vi "USB2XXX_UART_WriteReadTest.vi"() -> ()   [LabVIEW 2010]
panel:
  in  "pConfig":T1={"BaudRate"=19200, "WordLength"=0, "StopBits"=0, "Parity"=0, "TEPolarity"=0}
  out "Readed Data Num":i32
  out "Read Data(Hex)":string
  in  "Write Data(Hex)":string="11 22 33 44 55 66 77 88"
  in  "Channel Index":u8(ring) items=["UART0", "UART1"]
  in  "Device Index":i32(ring) items=["0", "1", "2", "3", "4", "5"]
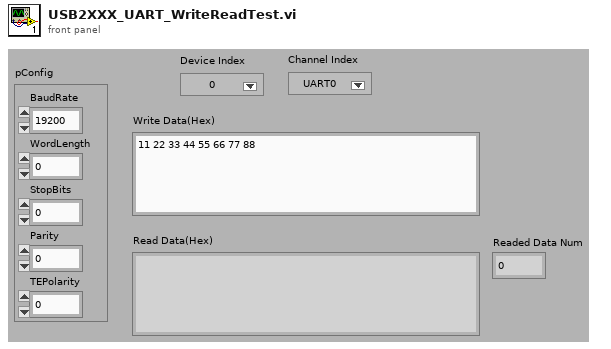
[diagram p1: front panel]
types:
  T1 = cluster{"BaudRate":u32, "WordLength":u8, "StopBits":u8, "Parity":u8, "TEPolarity":u8}
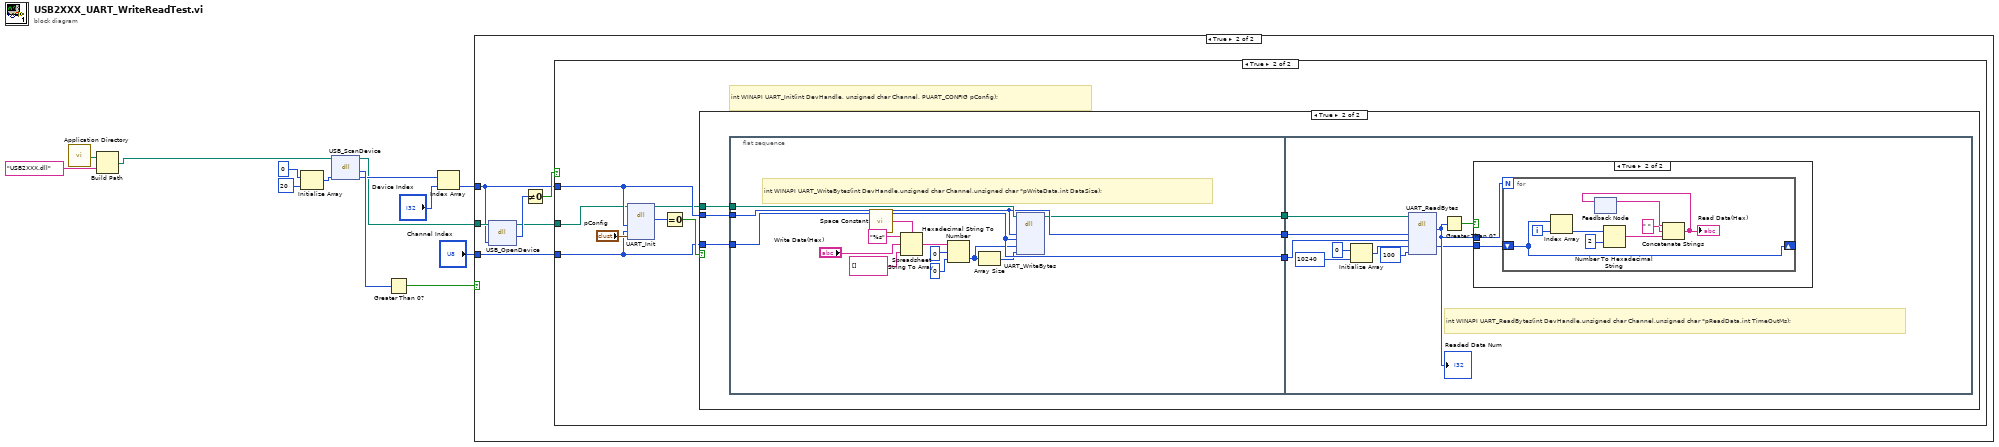
[diagram p0: block diagram]
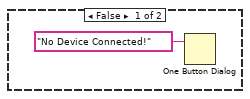
[diagram p2: hidden frame]
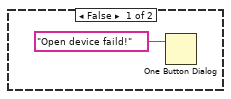
[diagram p3: hidden frame]
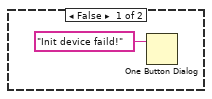
[diagram p4: hidden frame]
diagram:
  n1 = call <vilib>:"Application Directory.vi"() -> ("Application Directory"=w2:path)
  n2 = Build Path(base path=w2, name or relative path="USB2XXX.dll") -> (appended path=w1:path)
  n3 = Initialize Array(0, 20 ("dimension size")) -> (w11:i32[])
  n4 = dll-call lib="E:/OtherWork/STM32/USB2XXX_Example/examples/Labview/PublicFiles/USB2XXX.dll" fn="USB_ScanDevice"(path in=w1, "pDevNum"=w11) -> (path out=w6:path, "return type"=w10:i32, "pDevNum"=w9:i32[])  [unwired: 2 in, 1 out]
  n5 = Greater Than 0?(x=w10) -> (x > 0?=w7:bool)
  n6 = Index Array(array=w9, index="Device Index") -> (element=w5:i32)
  n7 = case shown="True" w7 {
    tunnel: w6 -> [_ w20]
    tunnel: w5 -> [_ w16]
    tunnel: "Channel Index" -> [_ w15]
    frame False {
      n8 = One Button Dialog(message="No Device Connected!") -> ()  [unwired: 1 in, 1 out]
    }
    frame True {
      n9 = dll-call lib="E:/OtherWork/STM32/USB2XXX_Example/examples/Labview/PublicFiles/USB2XXX.dll" fn="USB_OpenDevice"(path in=w20, "DevIndex"=w16) -> (path out=w17:path, "return type"=w19:u8)  [unwired: 3 in, 1 out]
      n10 = Not Equal To 0?(x=w19) -> (x != 0?=w18:bool)
      n11 = case shown="True" w18 {
        tunnel: w17 -> [_ w24]
        tunnel: w16 -> [_ w26]
        tunnel: w15 -> [_ w25]
        frame False {
          n12 = One Button Dialog(message="Open device faild!") -> ()  [unwired: 1 in, 1 out]
        }
        frame True {
          # "int WINAPI UART_Init(int DevHandle, unsigned char Channel, PUART_CONFIG pConfig);"
          n13 = dll-call lib="E:/OtherWork/STM32/USB2XXX_Example/sdk/api/Labview/USB2XXX.*" fn="UART_Init"(path in=w24, "DevHandle"=w26, "Channel"=w25, "pConfig"="pConfig") -> (path out=w23:path, "return type"=w22:i32)  [unwired: 5 in, 1 out]
          n14 = Equal To 0?(x=w22) -> (x = 0?=w28:bool)
          n15 = case shown="True" w28 {
            tunnel: w23 -> [_ w35]
            tunnel: w26 -> [_ w34]
            tunnel: w25 -> [_ w33]
            frame False {
              n16 = One Button Dialog(message="Init device faild!") -> ()  [unwired: 1 in, 1 out]
            }
            frame True {
              n17 = flat-sequence {
                tunnel: w35 -> [w41]
                tunnel: w34 -> [w40]
                tunnel: w33 -> [w39]
                tunnel: [w36] -> w32
                tunnel: [w40] -> w31
                tunnel: [w39] -> w30
                tunnel: w32 -> [w55]
                tunnel: w31 -> [w54]
                tunnel: w30 -> [w53]
                frame #0 {
                  # "int WINAPI UART_WriteBytes(int DevHandle,unsigned char Channel,unsigned char *pWriteData,int DataSize);"
                  n18 = call <vilib>:"Space Constant.vi"() -> ("String"=w44:string)
                  n19 = Spreadsheet String To Array(delimiter (Tab)=w44, format string="%s", spreadsheet string="Write Data(Hex)", array type (2D Dbl)=string[] []) -> (array=w47:string[])
                  n20 = Hexadecimal String To Number(string=w47, offset=0, default (0uL)=u8 0 ("default (0 U32)")) -> (number=w38:u8[])  [unwired: 1 out]
                  n21 = Array Size(array=w38) -> (size(s)=w37:i32)
                  n22 = dll-call lib="E:/OtherWork/STM32/USB2XXX_Example/sdk/api/Labview/USB2XXX.*" fn="UART_WriteBytes"(path in=w41, "DevHandle"=w40, "Channel"=w39, "pWriteData"=w38, "DataSize"=w37) -> (path out=w36:path)  [unwired: 7 in, 1 out]
                }
                frame #1 {
                  # "int WINAPI UART_ReadBytes(int DevHandle,unsigned char Channel,unsigned char *pReadData,int TimeOutMs);"
                  n23 = Initialize Array(u8 0 ("element"), 10240 ("dimension size")) -> (w52:u8[])
                  n24 = dll-call lib="E:/OtherWork/STM32/USB2XXX_Example/sdk/api/Labview/USB2XXX.*" fn="UART_ReadBytes"(path in=w55, "DevHandle"=w54, "Channel"=w53, "pReadData"=w52, "TimeOutMs"=100) -> ("return type"=w50:i32, "pReadData"=w49:u8[])  [unwired: 5 in, 2 out]
                  "Readed Data Num" <- w50
                  n25 = Greater Than 0?(x=w50) -> (x > 0?=w58:bool)
                  n26 = case shown="True" w58 {
                    tunnel: w50 -> [_ w60]
                    tunnel: w49 -> [_ w59]
                    frame False {
                    }
                    frame True {
                      n27 = for {
                        N: w60 -> [_]
                        shift-right: [w61] -> _
                        shift-left: w59 -> [w61]
                        i -> [w68]
                        n28 = Index Array(array=w61, index=w68) -> (element=w67:u8)
                        n29 = feedback #1() -> (w65:string)  [unwired: 1 in]
                        n30 = Number To Hexadecimal String(1:i16 2 ("width (-)"), 2:w67) -> (0:w63:string)
                        n31 = Concatenate Strings(w65, " " ("string"), w63) -> (w62:string)
                        "Read Data(Hex)" <- w62
                        n32 = feedback-in #1(w62) -> ()
                      }
                    }
                  }
                }
              }
            }
          }
        }
      }
    }
  }
